vi "Init Slider Boundaries.vi"(11 "DofType":T1) -> (1 "Unit Labels":string[](array[string]), 2 "Dof Labels":string[](array[string]), 3 "Boundaries":cluster{"[0]":dbl, "[1]":dbl}[](array[cluster]))   [LabVIEW 2013]
uses:
  Data Access Objects/Limits/DofTypes.ctl
  Data Access Objects/Metadata/Persistant DAO Actions.ctl
panel:
  in  "Cart Increment Labels":string[](array[string])=["Increment Dx", "Increment Dy", "Increment Dz", "Increment Rx", "Increment Ry", "Increment \n\n\n\n\n\n\n\n\n\n\n\n\n\n\n\n\n\n\n\n\n\n\n\n\n\n\n\n\nIncrement Rz\n\n"]
  in  "Act Increment Labels":string[](array[string])=["Increment X1", "Increment X2", "Increment Y1", "Increment Z1", "Increment Z2", "Increment Z3"]
  in  "Cart Displacement Labels":string[](array[string])=["Displacement X", "Displacement Y", "Displacement Z", "Rotation X", "Rotation Y", "Rotation Z"]
  in  "Cart Force Labels":string[](array[string])=["Force X", "Force Y", "Force Z", "Moment X", "Moment Y", "Moment Z"]
  in  "Act Force Labels":string[](array[string])=["Force X1", "Force X2", "Force Y1", "Force Z1", "Force Z2", "Force Z3"]
  in  "Act Disp Labels":string[](array[string])=["Displacement X1", "Displacement X2", "Displacement Y1", "Displacement Z1", "Displacement Z2", "Displacement Z3"]
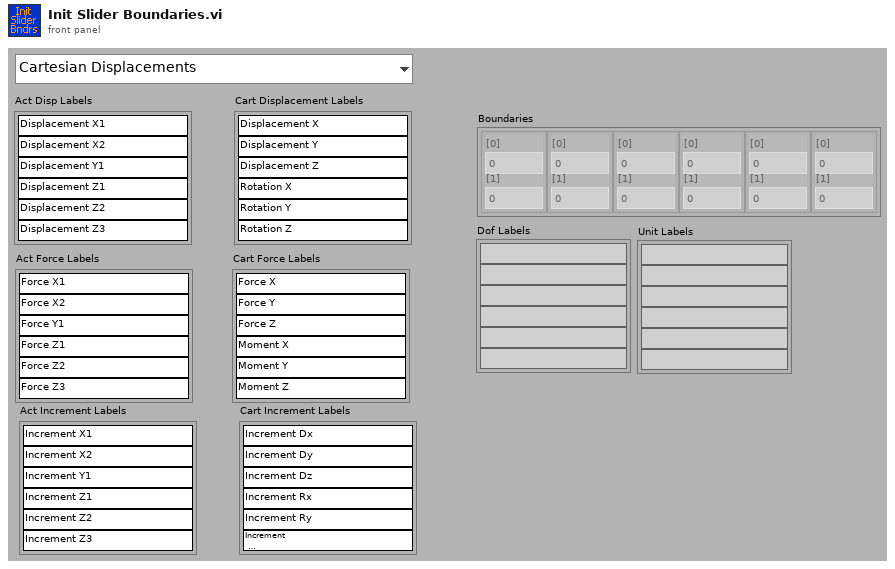
[diagram p1: front panel]
types:
  T1 = typedef "DofTypes.ctl" = enum16{"Cartesian Displacements", "Cartesian Forces & Moments", "Actuator Displacements", "Actuator Forces", "Cartesian Increments", "Actuator Increments"}
  T2 = typedef "Persistant DAO Actions.ctl" = enum16{"Init", "Get", "Set", "Load", "Save"}
  T3 = typedef "Limit Boundary Parameters.ctl" = cluster{"Lower":dbl, "Upper":dbl, "Label":string}
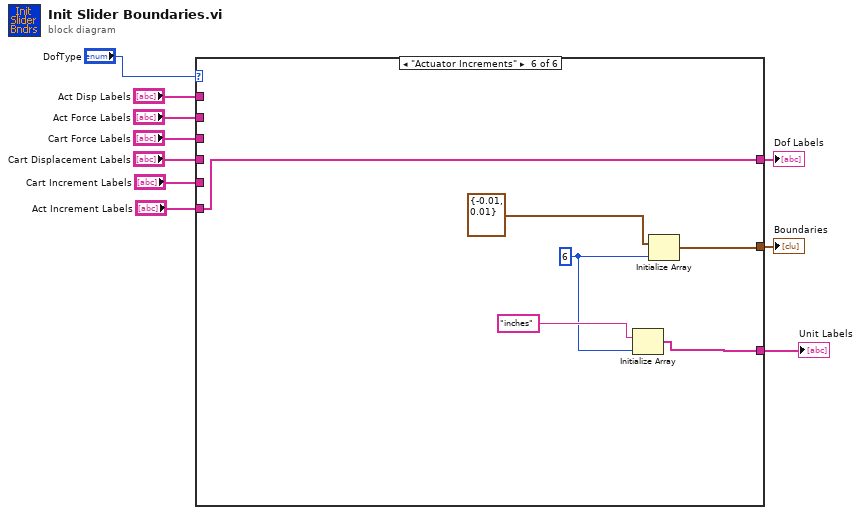
[diagram p0: block diagram]
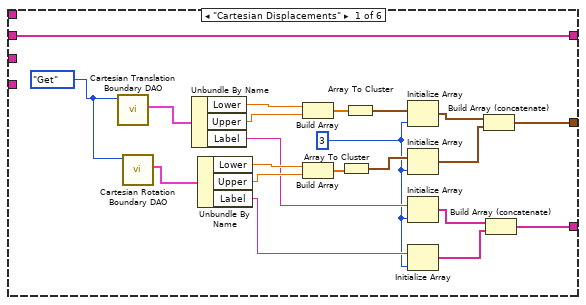
[diagram p2: hidden frame]
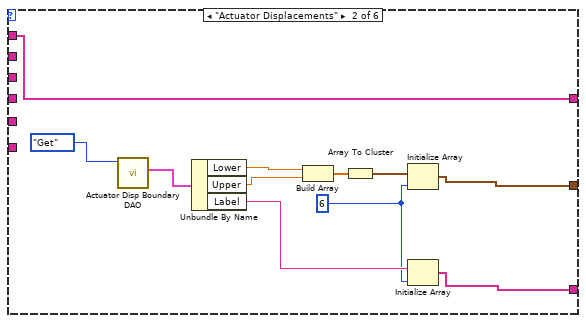
[diagram p3: hidden frame]
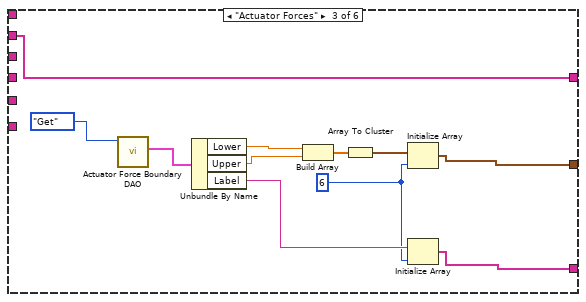
[diagram p4: hidden frame]
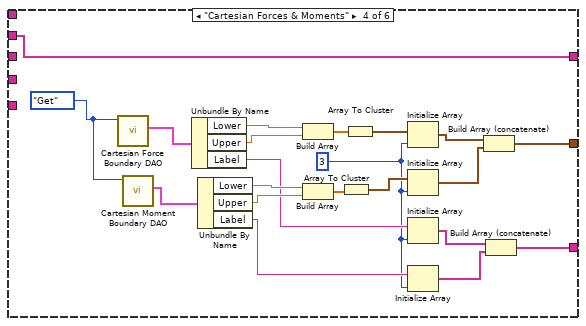
[diagram p5: hidden frame]
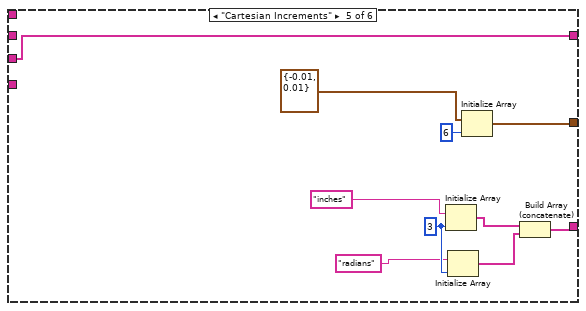
[diagram p6: hidden frame]
diagram:
  n1 = case shown="\"Actuator Increments\"" "DofType" {
    tunnel: "Act Disp Labels" -> [_ w32 _ _ _ _]
    tunnel: "Act Force Labels" -> [_ _ w43 _ _ _]
    tunnel: "Cart Force Labels" -> [_ _ _ w54 _ _]
    tunnel: "Cart Displacement Labels" -> [w11 _ _ _ _ _]
    tunnel: [w15 w33 w44 w58 w75 w88] -> w3
    tunnel: [w12 w34 w45 w55 w80 w86] -> w4
    tunnel: [w11 w32 w43 w54 w84 w85] -> w5
    tunnel: "Cart Increment Labels" -> [_ _ _ _ w84 _]
    tunnel: "Act Increment Labels" -> [_ _ _ _ _ w85]
    frame "Cartesian Displacements" {
      w18 = 3 ("dimension size")
      w31 = Persistant_DAO_Actions."Get" ("Actions")
      n2 = call "Cartesian Translation Boundary DAO.vi"("Actions"=w31) -> ("Limit Boundary Parameters Out"=w30:T3)  [unwired: 8 in, 2 out]
      n3 = call "Cartesian Rotation Boundary DAO.vi"("Actions"=w31) -> ("Limit Boundary Parameters Out"=w29:T3)  [unwired: 8 in, 2 out]
      n4 = Unbundle By Name(w30) -> ("Lower"=w28:dbl, "Upper"=w27:dbl, "Label"=w20:string)
      n5 = Unbundle By Name(w29) -> ("Lower"=w26:dbl, "Upper"=w25:dbl, "Label"=w19:string)
      n6 = Build Array(w28, w27) -> (w24:dbl[])
      n7 = Build Array(w26, w25) -> (w22:dbl[])
      n8 = Array To Cluster(array=w22) -> (cluster=w21:cluster{"[0]":dbl, "[1]":dbl})
      n9 = Array To Cluster(array=w24) -> (cluster=w23:cluster{"[0]":dbl, "[1]":dbl})
      n10 = Initialize Array(w23, w18) -> (w17:cluster{"[0]":dbl, "[1]":dbl}[])
      n11 = Initialize Array(w21, w18) -> (w16:cluster{"[0]":dbl, "[1]":dbl}[])
      n12 = Initialize Array(w20, w18) -> (w14:string[])
      n13 = Initialize Array(w19, w18) -> (w13:string[])
      n14 = Build Array (concatenate)(w17, w16) -> (w15:cluster{"[0]":dbl, "[1]":dbl}[])
      n15 = Build Array (concatenate)(w14, w13) -> (w12:string[])
    }
    frame "Actuator Displacements" {
      w35 = 6 ("dimension size")
      n16 = call "Actuator Disp Boundary DAO.vi"("Actions"=Persistant_DAO_Actions."Get") -> ("Limit Boundary Parameters Out"=w41:T3)  [unwired: 8 in, 2 out]
      n17 = Unbundle By Name(w41) -> ("Lower"=w40:dbl, "Upper"=w39:dbl, "Label"=w36:string)
      n18 = Build Array(w40, w39) -> (w38:dbl[])
      n19 = Array To Cluster(array=w38) -> (cluster=w37:cluster{"[0]":dbl, "[1]":dbl})
      n20 = Initialize Array(w37, w35) -> (w33:cluster{"[0]":dbl, "[1]":dbl}[])
      n21 = Initialize Array(w36, w35) -> (w34:string[])
    }
    frame "Actuator Forces" {
      w46 = 6 ("dimension size")
      n22 = call "Actuator Force Boundary DAO.vi"("Actions"=Persistant_DAO_Actions."Get") -> ("Limit Boundary Parameters Out"=w52:T3)  [unwired: 8 in, 2 out]
      n23 = Unbundle By Name(w52) -> ("Lower"=w51:dbl, "Upper"=w50:dbl, "Label"=w47:string)
      n24 = Build Array(w51, w50) -> (w49:dbl[])
      n25 = Array To Cluster(array=w49) -> (cluster=w48:cluster{"[0]":dbl, "[1]":dbl})
      n26 = Initialize Array(w48, w46) -> (w44:cluster{"[0]":dbl, "[1]":dbl}[])
      n27 = Initialize Array(w47, w46) -> (w45:string[])
    }
    frame "Cartesian Forces & Moments" {
      w61 = 3 ("dimension size")
      w74 = Persistant_DAO_Actions."Get" ("Actions")
      n28 = call "Cartesian Force Boundary DAO.vi"("Actions"=w74) -> ("Limit Boundary Parameters Out"=w73:T3)  [unwired: 8 in, 2 out]
      n29 = call "Cartesian Moment Boundary DAO.vi"("Actions"=w74) -> ("Limit Boundary Parameters Out"=w72:T3)  [unwired: 8 in, 2 out]
      n30 = Unbundle By Name(w73) -> ("Lower"=w71:dbl, "Upper"=w70:dbl, "Label"=w63:string)
      n31 = Unbundle By Name(w72) -> ("Lower"=w69:dbl, "Upper"=w68:dbl, "Label"=w62:string)
      n32 = Build Array(w71, w70) -> (w67:dbl[])
      n33 = Build Array(w69, w68) -> (w65:dbl[])
      n34 = Array To Cluster(array=w65) -> (cluster=w64:cluster{"[0]":dbl, "[1]":dbl})
      n35 = Array To Cluster(array=w67) -> (cluster=w66:cluster{"[0]":dbl, "[1]":dbl})
      n36 = Initialize Array(w66, w61) -> (w60:cluster{"[0]":dbl, "[1]":dbl}[])
      n37 = Initialize Array(w64, w61) -> (w59:cluster{"[0]":dbl, "[1]":dbl}[])
      n38 = Initialize Array(w63, w61) -> (w57:string[])
      n39 = Initialize Array(w62, w61) -> (w56:string[])
      n40 = Build Array (concatenate)(w60, w59) -> (w58:cluster{"[0]":dbl, "[1]":dbl}[])
      n41 = Build Array (concatenate)(w57, w56) -> (w55:string[])
    }
    frame "Cartesian Increments" {
      w82 = 3 ("dimension size")
      n42 = Initialize Array("inches", w82) -> (w79:string[])
      n43 = Initialize Array("radians", w82) -> (w78:string[])
      n44 = Initialize Array(cluster{"[0]":dbl, "[1]":dbl} {"[0]"=-0.01, "[1]"=0.01}, 6 ("dimension size")) -> (w75:cluster{"[0]":dbl, "[1]":dbl}[])
      n45 = Build Array (concatenate)(w79, w78) -> (w80:string[])
    }
    frame "Actuator Increments" {
      w87 = 6 ("dimension size")
      n46 = Initialize Array("inches", w87) -> (w86:string[])
      n47 = Initialize Array(cluster{"[0]":dbl, "[1]":dbl} {"[0]"=-0.01, "[1]"=0.01}, w87) -> (w88:cluster{"[0]":dbl, "[1]":dbl}[])
    }
  }
  "Dof Labels" <- w5
  "Unit Labels" <- w4
  "Boundaries" <- w3
